vi "Get Callback Events.vi"(11 "MyEventGrid in":refnum<class "MyEventGrid.lvclass">) -> (2 "Callback Events":T1, 3 "MyEventGrid out":refnum<class "MyEventGrid.lvclass">)   [LabVIEW 2023, in "MyEventGrid.lvclass"]
uses:
  MyEventGrid.lvclass
  source/Cells/Cell Context/Cell Context.lvclass
  MyEventGrid.lvclass/MyEventGrid.ctl
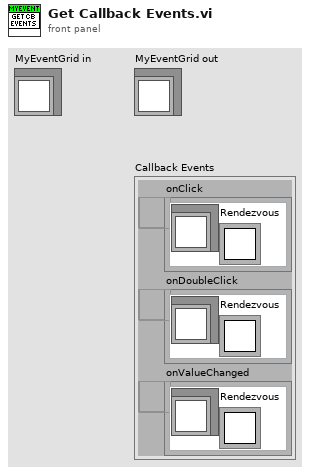
[diagram p1: front panel]
types:
  T1 = cluster{"onClick":refnum<user-event>, "onDoubleClick":refnum<user-event>, "onValueChanged":refnum<user-event>}
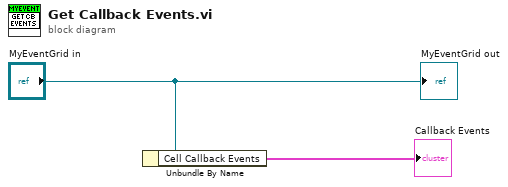
[diagram p0: block diagram]
diagram:
  n1 = Unbundle By Name("MyEventGrid in") -> ("Cell Callback Events"=→"Callback Events":T1)
  "MyEventGrid out" <- "MyEventGrid in"
